vi "PC_Pub_imgFile execution.vi"() -> ()   [LabVIEW 2018]
uses:
  <vilib>/Utility/miscctls.llb/LVRowAndColumnTypeDef.ctl
  <vilib>/nisyscfg/nisyscfg.lvlib
  <resource>/objmgr/nisysapi.rc
  <vilib>/nisyscfg/Close (System).vi
  <vilib>/nisyscfg/Get Installed Components.vi
  QMH/QMH.lvclass
  PC_Pub_imgFile.lvclass
  ProgressBar/ProgressBar.lvclass
  <vilib>/nisyscfg/Create System Image (File).vi
panel:
  in  "Progress":i32(slide) caption="imgDeploy" scale=0.0..100.0
  in  "Retrieve":bool
  in  "Application Image List":string[][](table)
  in  "Deploy":bool
  in  "Target":string(combo)
  out "Current Version":string
  in  "New Version":string
  in  "Description":string
  in  "Title":string
  in  "Image Storage Path":path
  out "Abort":bool
  in  "progressCaption":string
  out "error out":errorcluster
  # "Application Image Properties"
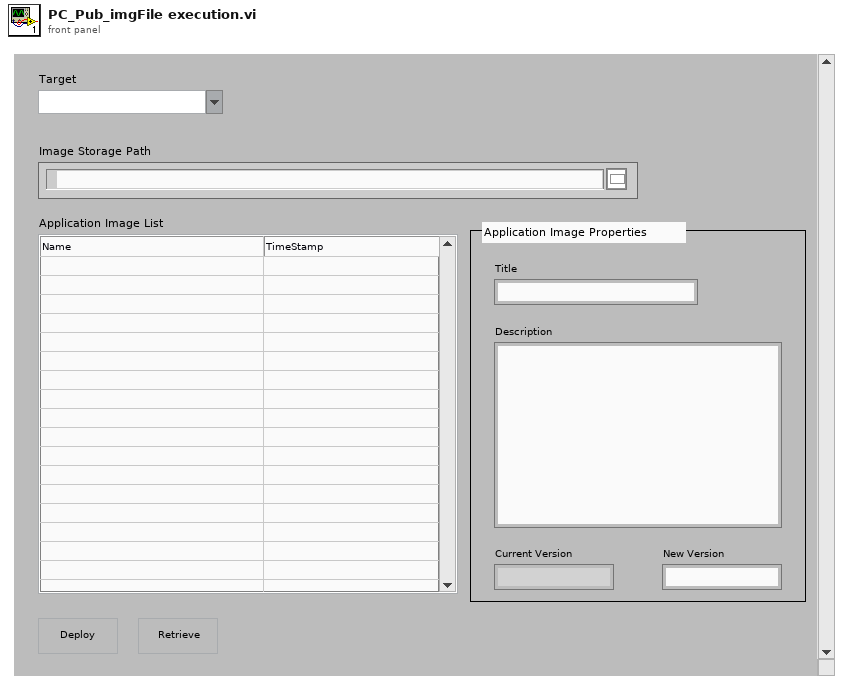
[diagram p1: front panel]
types:
  T1 = typedef "LVRowAndColumnTypeDef.ctl" = cluster{"Row":i32, "Column":i32}
  T2 = cluster{"thisVIRefnum":refnum<vi>, "progressBarRefnum":refnum<vi>, "progressCaption":refnum<vi>}
  T3 = cluster{"Target":refnum<vi>, "Image Storage Path":refnum<vi>, "Pane":refnum<vi>, "Application Image List":refnum<vi>, "Properties":cluster{"Title":refnum<vi>, "Description":refnum<vi>, "Current Version":refnum<vi>, "New Version":refnum<vi>, "id":string}}
  T4 = cluster{"Title":refnum<vi>, "Description":refnum<vi>, "Current Version":refnum<vi>, "New Version":refnum<vi>, "id":string}
  T5 = enum8{"Enabled", "Disabled", "Disabled and Grayed Out"}
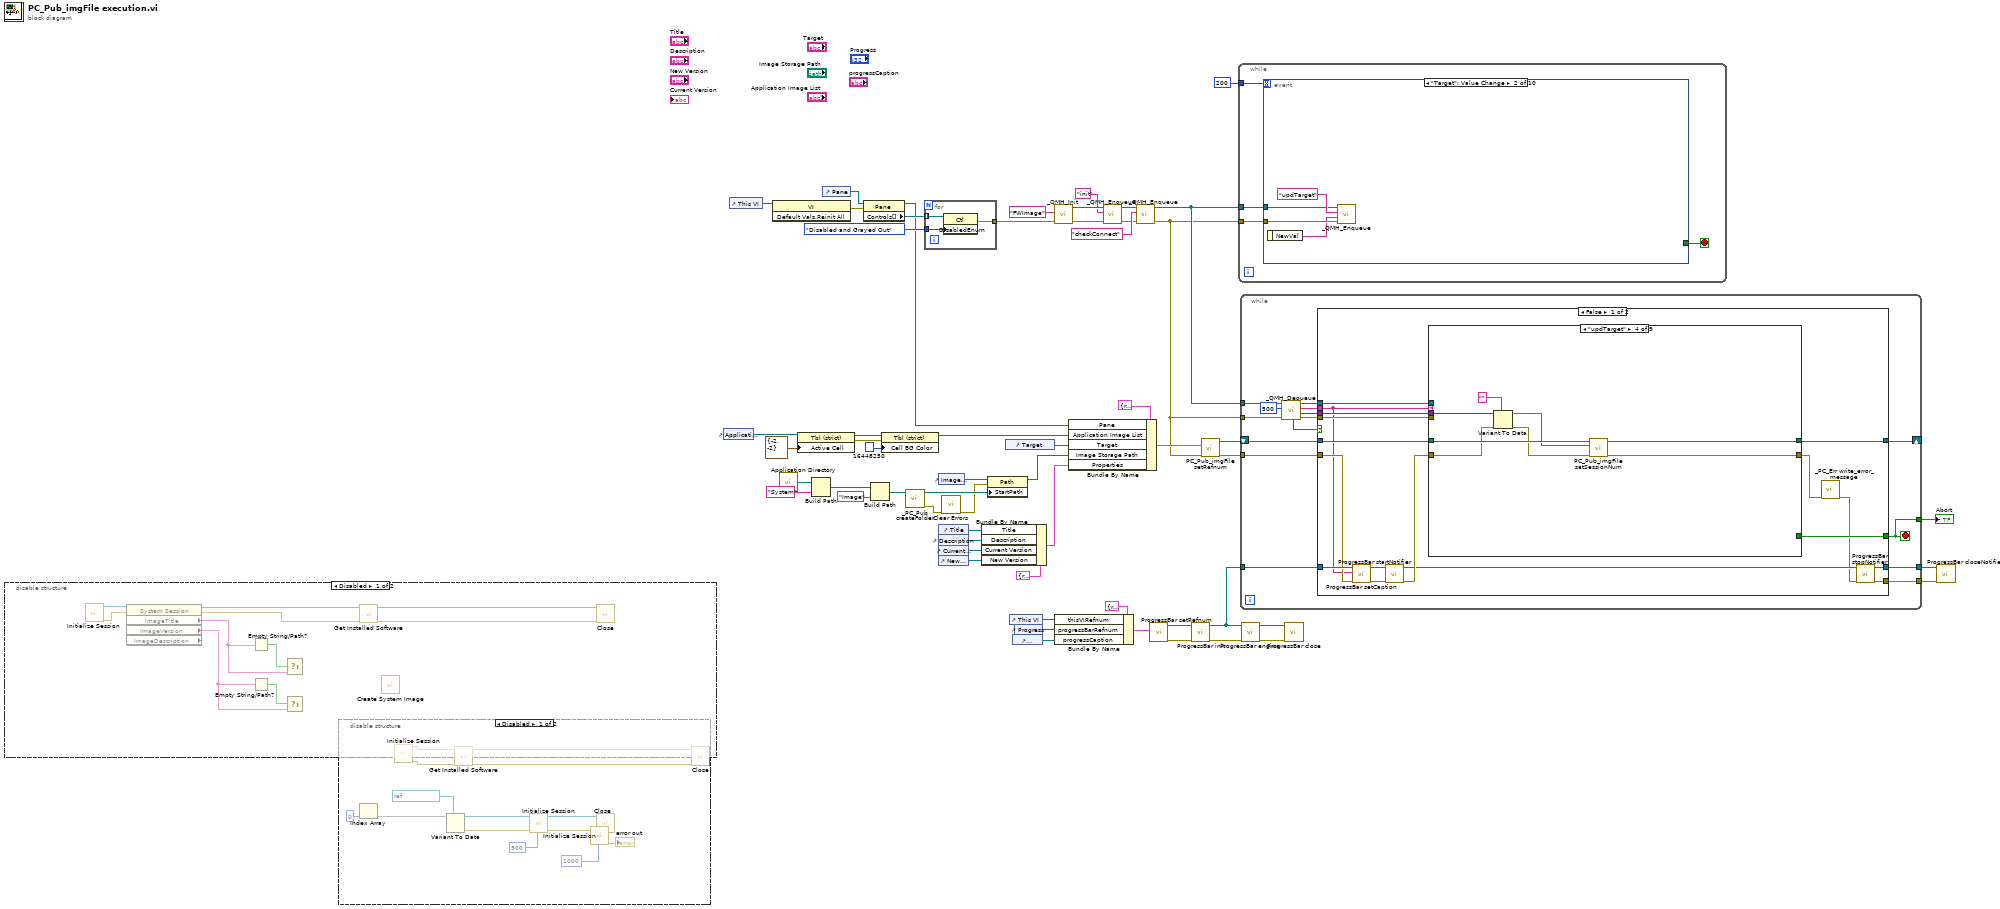
[diagram p0: block diagram]
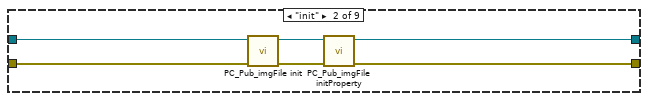
[diagram p3: hidden frame]
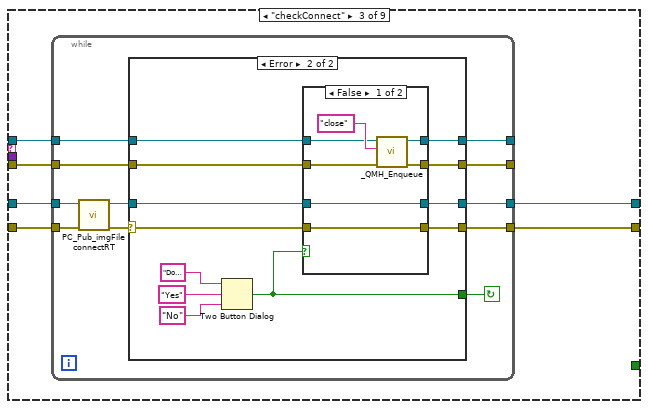
[diagram p4: hidden frame]
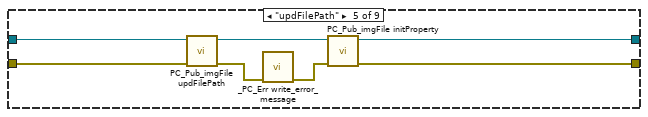
[diagram p7: hidden frame]
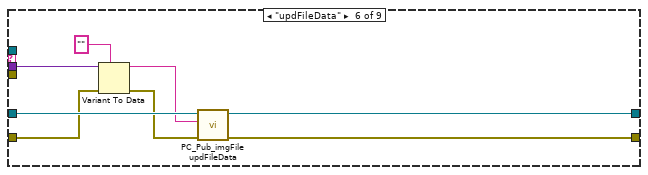
[diagram p8: hidden frame]
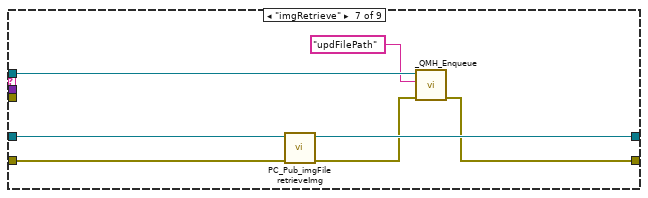
[diagram p9: hidden frame]
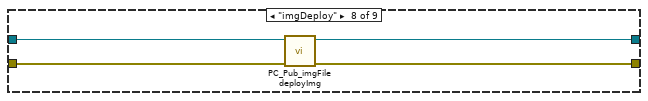
[diagram p10: hidden frame]
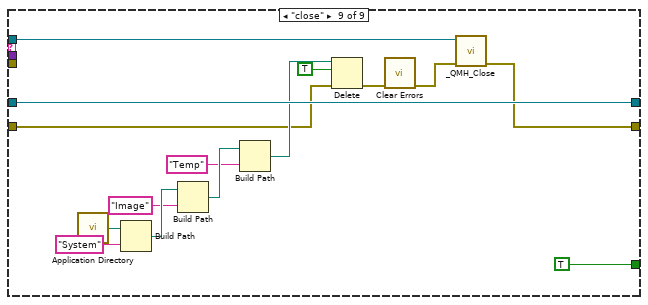
[diagram p11: hidden frame]
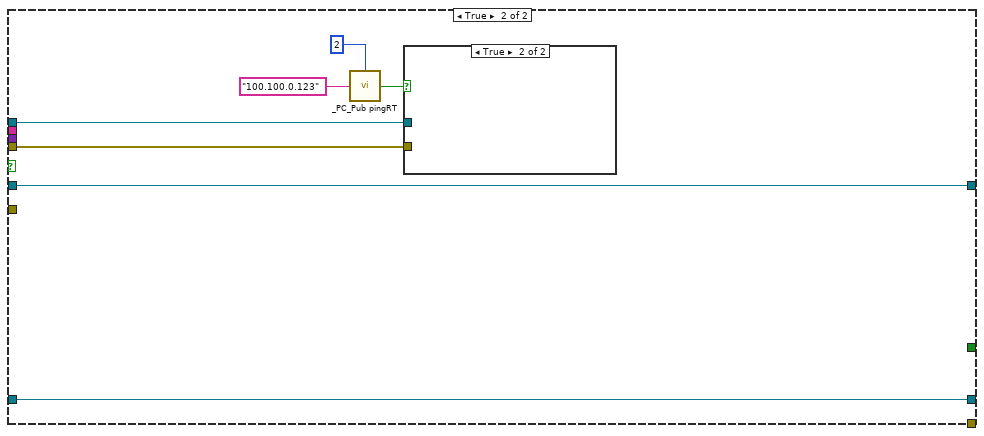
[diagram p12: hidden frame]
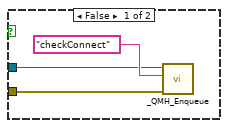
[diagram p13: hidden frame]
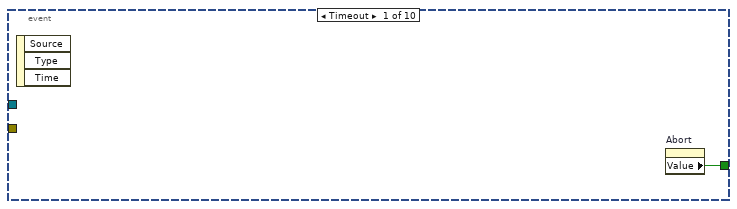
[diagram p14: hidden frame]
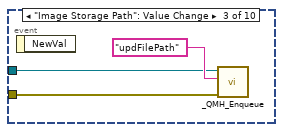
[diagram p15: hidden frame]
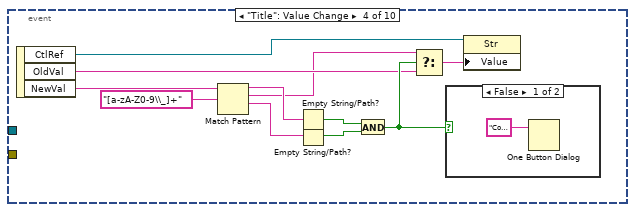
[diagram p16: hidden frame]
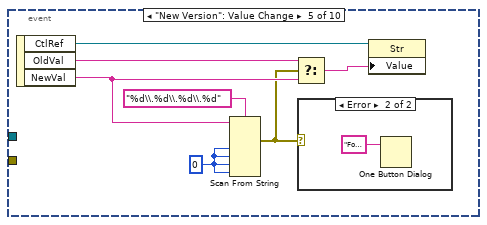
[diagram p18: hidden frame]
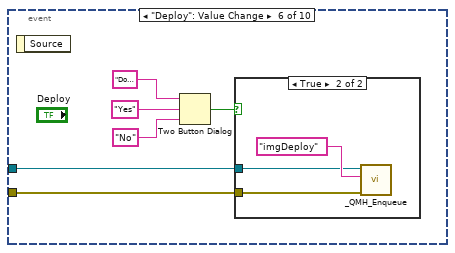
[diagram p20: hidden frame]
diagram:
  n1 = disable-structure shown="Disabled" {
    frame Disabled {
      n2 = call <vilib>:"Initialize Session.vi"() -> ("error out"=w63:errorcluster, "Session out"=w64:refnum<k21>, "Target (localhost)"=w65:refnum<k21>)  [unwired: 9 in]
      n3 = property class="System Session" props=["ImageTitle", "ImageVersion", "ImageDescription"](reference=w64, error in=w63) -> (reference out=w62:refnum<k21>, error out=w61:errorcluster, "ImageTitle"=w69:string, "ImageVersion"=w71:string)  [unwired: 1 out]
      n4 = Empty String/Path?(string/path=w69) -> (empty?=w68:bool)
      n5 = Empty String/Path?(string/path=w71) -> (empty?=w70:bool)
      n6 = Select(s=w68, f=w69) -> (t=w66:string)  [unwired: 1 out]
      n7 = Select(s=w70, f=w71) -> (t=w67:string)  [unwired: 1 out]
      n8 = call-poly <vilib>:"Get Installed Software.vi"("error in (no error)"=w61, "Session in"=w62) -> ("error out"=w59:errorcluster, "Session out"=w60:refnum<k21>)  [unwired: 7 in, 1 out]
      n9 = call-poly <vilib>:"Create System Image.vi"() -> ()  [unwired: 9 in, 3 out]
      n10 = call-poly <vilib>:"Close.vi"("error in (no error)"=w59, "Session in"=w60) -> ()  [unwired: 9 in, 1 out]
    }
    frame Enabled {
    }
  }
  n11 = disable-structure shown="Disabled" {
    frame Disabled {
      n12 = Index Array(index=0) -> (element=w77)  [unwired: 1 in]
      n13 = call <vilib>:"Initialize Session.vi"() -> ("error out"=w84:errorcluster, "Session out"=w85:refnum<k21>, "Target (localhost)"=w80:refnum<k21>)  [unwired: 9 in]
      n14 = Variant To Data(type=refnum<k21> "localhost" ("Target (localhost)"), Variant=w77) -> (data=w76:refnum<k21>, error out=w75:errorcluster)  [unwired: 1 in]
      n15 = call-poly <vilib>:"Get Installed Software.vi"("error in (no error)"=w84, "Session in"=w85) -> ("error out"=w86:errorcluster, "Session out"=w87:refnum<k21>)  [unwired: 7 in, 1 out]
      n16 = call <vilib>:"Initialize Session.vi"("Connect Timeout (4000 ms)"=u32 500, "error in (no error)"=w75, "Target (localhost)"=w76) -> ("error out"=w72:errorcluster, "Session out"=w73:refnum<k21>)  [unwired: 7 in]
      n17 = call <vilib>:"Initialize Session.vi"("Connect Timeout (4000 ms)"=u32 1000) -> ("error out"=→"error out":errorcluster, "Target (localhost)"=w82:refnum<k21>)  [unwired: 8 in, 1 out]
      n18 = call-poly <vilib>:"Close.vi"("error in (no error)"=w72, "Session in"=w73) -> ()  [unwired: 9 in, 1 out]
      n19 = call-poly <vilib>:"Close.vi"("error in (no error)"=w86, "Session in"=w87) -> ()  [unwired: 9 in, 1 out]
    }
    frame Enabled {
    }
  }
  n20 = control-ref of="Application Image List"() -> (w5:refnum<vi>)
  n21 = control-ref of="This VI"() -> (w41:refnum<vi>)
  n22 = invoke class="VI" method="Default Vals.Reinit All"(reference=w41) -> (error out=w40:errorcluster)  [unwired: 2 in, 2 out]
  n23 = call <vilib>:"Application Directory.vi"() -> ("Application Directory"=w38:path)
  n24 = property class="Tbl (strict)"(reference=w5, "Active Cell"=T1 {"Row"=-2, "Column"=-2} ("Active Cell:Active Cell")) -> (reference out=w8:refnum<vi>, error out=w7:errorcluster)  [unwired: 1 in]
  n25 = Build Path(base path=w38, name or relative path="System") -> (appended path=w36:path)
  n26 = control-ref of="Pane"() -> (w57:refnum<vi>)
  n27 = property class="Pane"(reference=w57, error in=w40) -> (reference out=w3:refnum<vi>, "Controls[]"=w56:refnum<vi>[])  [unwired: 1 out]
  n28 = Build Path(base path=w36, name or relative path="Image") -> (appended path=w34:path)
  n29 = property class="Tbl (strict)"(reference=w8, error in=w7, "Cell BG Color"=u32 16448250) -> (reference out=w4:refnum<vi>)  [unwired: 1 out]
  n30 = call "_PC_Pub createFolder.vi"("path (use dialog)"=w34) -> ("error out"=w32:errorcluster, "created path"=w33:path)  [unwired: 9 in]
  n31 = for {
    tunnel: w56 -> [w90] mode=indexing
    tunnel: T5."Disabled and Grayed Out" ("Disabled") -> [w89]
    tunnel: [w88] -> w45
    n32 = property class="Ctl"(reference=w90, "DisabledEnum"=w89) -> (error out=w88:errorcluster)  [unwired: 1 in, 1 out]
  }
  n33 = control-ref of="Title"() -> (w54:refnum<vi>)
  n34 = control-ref of="Description"() -> (w53:refnum<vi>)
  n35 = control-ref of="Current Version"() -> (w52:refnum<vi>)
  n36 = control-ref of="New Version"() -> (w51:refnum<vi>)
  n37 = control-ref of="Image Storage Path"() -> (w43:refnum<vi>)
  n38 = call <vilib>:"Clear Errors.vi"("error in (no error)"=w32) -> ("error out"=w31:errorcluster)  [unwired: 5 in, 1 out]
  n39 = Bundle By Name(cluster=T4 {"Title"=refnum, "Description"=refnum, "Current Version"=refnum, "New Version"=refnum, "id"=""} ("Properties"), "Title"=w54, "Description"=w53, "Current Version"=w52, "New Version"=w51) -> (w42:T4)
  n40 = property class="Path"(reference=w43, error in=w31, "StartPath"=w33) -> (reference out=w39:refnum<vi>)  [unwired: 1 out]
  n41 = control-ref of="Target"() -> (w44:refnum<vi>)
  n42 = control-ref of="This VI"() -> (w17:refnum<vi>)
  n43 = control-ref of="progressCaption"() -> (w15:refnum<vi>)
  n44 = control-ref of="Progress"() -> (w16:refnum<vi>)
  n45 = call "_QMH_Init.vi"("error in (no error)"=w45, "name (unnamed)"="FWImage") -> ("error out"=w29:errorcluster, "QMH out"=w30:refnum<class "QMH.lvclass">)  [unwired: 8 in]
  n46 = Bundle By Name(cluster=T2 {"thisVIRefnum"=refnum, "progressBarRefnum"=refnum, "progressCaption"=refnum} ("refnum"), "thisVIRefnum"=w17, "progressBarRefnum"=w16, "progressCaption"=w15) -> (w14:T2)
  n47 = Bundle By Name(cluster=T3 {"Target"=refnum, "Image Storage Path"=refnum, "Pane"=refnum, "Application Image List"=refnum, "Properties"={"Title"=refnum, "Description"=refnum, "Current Version"=refnum, "New Version"=refnum, "id"=""}} ("refnum"), "Pane"=w3, "Application Image List"=w4, "Target"=w44, "Image Storage Path"=w39, "Properties"=w42) -> (w46:T3)
  n48 = call "_QMH_Enqueue.vi"("error in (no error)"=w29, "Msg"="init", "QMH in"=w30) -> ("error out"=w25:errorcluster, "QMH out"=w26:refnum<class "QMH.lvclass">)  [unwired: 7 in]
  n49 = call "_QMH_Enqueue.vi"("error in (no error)"=w25, "Msg"="checkConnect", "QMH in"=w26) -> ("error out"=w23:errorcluster, "QMH out"=w24:refnum<class "QMH.lvclass">)  [unwired: 7 in]
  n50 = call "ProgressBar setRefnum.vi"("refnum"=w14) -> ("error out"=w21:errorcluster, "ProgressBar out"=w22:refnum<class "ProgressBar.lvclass">)  [unwired: 9 in]
  n51 = call "ProgressBar init.vi"("error in (no error)"=w21, "ProgressBar in"=w22) -> ("error out"=w19:errorcluster, "ProgressBar out"=w20:refnum<class "ProgressBar.lvclass">)  [unwired: 8 in]
  n52 = call "PC_Pub_imgFile setRefnum.vi"("error in (no error)"=w23, "refnum"=w46) -> ("error out"=w48:errorcluster, "imgFile out"=w49:refnum<class "PC_Pub_imgFile.lvclass">)  [unwired: 8 in]
  n53 = while {
    tunnel: w24 -> [w94]
    tunnel: w23 -> [w93]
    tunnel: 200 -> [w91]
    stop <- w92 stop-if-true
    n54 = event shown="[1] \"Target\": Value Change" {
      selector: _ -> [_ _ _ _ _ _ _ _ _ _]
      dyn-events: _ -> [_ _ _ _ _ _ _ _ _ _]
      timeout: w91 -> [_ _ _ _ _ _ _ _ _ _]
      tunnel: w94 -> [_ w98 w101 _ _ w124 w134 _ w149 w165]
      tunnel: w93 -> [_ w97 w100 _ _ w123 w133 _ w148 w164]
      tunnel: [w95 _ _ _ _ _ _ _ _ TRUE] -> w92
      event Timeout {
        n55 = event-data() -> ()  [unwired: 1 in, 3 out]
        n56 = property on="Abort" class="Bool (strict)"() -> ("Value"=w95:bool)  [unwired: 2 in, 2 out]
      }
      event "Target": Value Change {
        n57 = event-data() -> ("NewVal"=w96:string)  [unwired: 1 in]
        n58 = call "_QMH_Enqueue.vi"("error in (no error)"=w97, "Data"=w96, "Msg"="updTarget", "QMH in"=w98) -> ()  [unwired: 6 in, 2 out]
      }
      event "Image Storage Path": Value Change {
        n59 = event-data() -> ()  [unwired: 1 in, 1 out]
        n60 = call "_QMH_Enqueue.vi"("error in (no error)"=w100, "Msg"="updFilePath", "QMH in"=w101) -> ()  [unwired: 7 in, 2 out]
      }
      event "Title": Value Change {
        n61 = event-data() -> ("CtlRef"=w107:refnum<vi>, "OldVal"=w104:string, "NewVal"=w112:string)  [unwired: 1 in]
        n62 = Match Pattern(string=w112, regular expression="[a-zA-Z0-9\\_]+") -> (before substring=w111:string, match substring=w103:string, after substring=w110:string)  [unwired: 1 in, 1 out]
        n63 = Empty String/Path?(string/path=w111) -> (empty?=w109:bool)
        n64 = Empty String/Path?(string/path=w110) -> (empty?=w108:bool)
        n65 = And(x=w109, y=w108) -> (x .and. y?=w105:bool)
        n66 = Select(t=w103, s=w105, f=w104) -> (s? t:f=w106:string)
        n67 = case shown="False" w105 {
          frame False {
            n68 = One Button Dialog(message="Contains incorrect characters") -> ()  [unwired: 1 in, 1 out]
          }
          frame True {
          }
        }
        n69 = property class="Str"(reference=w107, "Value"=w106) -> ()  [unwired: 1 in, 2 out]
      }
      event "New Version": Value Change {
        w121 = u16 0
        n70 = event-data() -> ("CtlRef"=w117:refnum<vi>, "OldVal"=w119:string, "NewVal"=w118:string)  [unwired: 1 in]
        n71 = Scan From String(format string="%d\\.%d\\.%d\\.%d", input string=w118, default 1=w121, default 2=w121, default 3=w121, default 4=w121) -> (error out=w115:errorcluster)  [unwired: 6 in, 2 out]
        n72 = Select(t=w119, s=w115, f=w118) -> (s? t:f=w116:string)
        n73 = case shown="Error" w115 {
          frame No Error {
          }
          frame Error {
            n74 = One Button Dialog(message="Format has error") -> ()  [unwired: 1 in, 1 out]
          }
        }
        n75 = property class="Str"(reference=w117, "Value"=w116) -> ()  [unwired: 1 in, 2 out]
      }
      event "Deploy": Value Change {
        n76 = event-data() -> ()  [unwired: 1 in, 1 out]
        n77 = Two Button Dialog(message="Do you want to deploy system image?", 1:"No" ("F button name (\"Cancel\")"), 2:"Yes" ("T button name (\"OK\")")) -> (T button?=w125:bool)
        n78 = case shown="True" w125 {
          tunnel: w124 -> [_ w130]
          tunnel: w123 -> [_ w129]
          frame False {
          }
          frame True {
            n79 = call "_QMH_Enqueue.vi"("error in (no error)"=w129, "Msg"="imgDeploy", "QMH in"=w130) -> ()  [unwired: 7 in, 2 out]
          }
        }
      }
      event "Retrieve": Value Change {
        n80 = event-data() -> ()  [unwired: 1 in, 1 out]
        n81 = Two Button Dialog(message="Do you want to retrieve system image?", 1:"No" ("F button name (\"Cancel\")"), 2:"Yes" ("T button name (\"OK\")")) -> (T button?=w135:bool)
        n82 = case shown="True" w135 {
          tunnel: w134 -> [_ w139]
          tunnel: w133 -> [_ w138]
          frame False {
          }
          frame True {
            n83 = call "_QMH_Enqueue.vi"("error in (no error)"=w138, "Msg"="imgRetrieve", "QMH in"=w139) -> ()  [unwired: 7 in, 2 out]
          }
        }
      }
      event "Application Image List": Mouse Down? {
        n84 = event-data() -> ("Mods.Double Click"=w142:bool)  [unwired: 1 in]
        n85 = Not(x=w142) -> (.not. x?=w141:bool)
        n86 = event-data("Discard?"=w141) -> ()  [unwired: 1 in, 1 out]
      }
      event "Application Image List": Mouse Down {
        n87 = event-data() -> ("CtlRef"=w156:refnum<vi>)  [unwired: 1 in]
        n88 = property class="Tbl (strict)"(reference=w156) -> (reference out=w155:refnum<vi>, "Value"=w152:string[][], "EditPos"=w153:T1)  [unwired: 1 in, 1 out]
        n89 = Unbundle By Name(w153) -> ("Row"=w143:i32)
        n90 = Index Array(array=w152, index (row)=w143) -> (element=w151:string[])  [unwired: 1 in]
        n91 = property class="Tbl (strict)"(reference=w155, "Key Focus"=FALSE) -> (reference out=w144:refnum<vi>)  [unwired: 1 in, 1 out]
        n92 = Index Array(array=w151, index=0) -> (element=w147:string)
        n93 = Empty String/Path?(string/path=w147) -> (empty?=w146:bool)
        n94 = case shown="False" w146 {
          tunnel: w149 -> [w162 _]
          tunnel: "updFileData" ("Msg") -> [w161 _]
          tunnel: w148 -> [w160 _]
          tunnel: w147 -> [w159 _]
          tunnel: w144 -> [w158 _]
          tunnel: w143 -> [w157 _]
          frame False {
            n95 = call "PC_Pub_imgFile markTableRow.vi"("Row"=w157, "tableRefNum"=w158) -> ()
            n96 = call "_QMH_Enqueue.vi"("error in (no error)"=w160, "Data"=w159, "Msg"=w161, "QMH in"=w162) -> ()  [unwired: 6 in, 2 out]
          }
          frame True {
          }
        }
      }
      event Panel Close {
        n97 = event-data() -> ()  [unwired: 1 in, 1 out]
        n98 = call "_QMH_Enqueue.vi"("error in (no error)"=w164, "Msg"="close", "QMH in"=w165) -> ()  [unwired: 7 in, 2 out]
      }
    }
  }
  n99 = while {
    tunnel: w24 -> [w178]
    tunnel: w48 -> [w180]
    shift-right: [w179] -> _
    shift-left: w49 -> [w181]
    tunnel: w23 -> [w175]
    tunnel: w20 -> [w170]
    tunnel: [w169] -> w13
    tunnel: [w168] -> w12
    tunnel: [w167] -> w1
    stop <- w167 stop-if-true
    n100 = call "_QMH_Dequeue.vi"("error in (no error)"=w175, "timeout in ms (-1)"=500, "QMH in"=w178) -> ("error out"=w173:errorcluster, "Data"=w171:variant, "Msg"=w174:string, "QMH out"=w176:refnum<class "QMH.lvclass">, "timed out?"=w172:bool)  [unwired: 3 in, 1 out]
    n101 = case shown="False" w172 {
      tunnel: w181 -> [w198 w302]
      tunnel: w180 -> [w187 _]
      tunnel: [w197 w302] -> w179
      tunnel: w176 -> [w196 w304]
      tunnel: w174 -> [w184 _]
      tunnel: w173 -> [w195 w303]
      tunnel: [w194 _] -> w167
      tunnel: w171 -> [w193 _]
      tunnel: w170 -> [w188 w301]
      tunnel: [w183 w301] -> w169
      tunnel: [w182 _] -> w168
      frame False {
        n102 = call "ProgressBar setCaption.vi"("error in (no error)"=w187, "newCaption"=w184, "ProgressBar in"=w188) -> ("error out"=w186:errorcluster, "ProgressBar out"=w185:refnum<class "ProgressBar.lvclass">)  [unwired: 7 in]
        n103 = call "ProgressBar startNotifier.vi"("error in (no error)"=w186, "ProgressBar in"=w185) -> ("error out"=w192:errorcluster, "ProgressBar out"=w191:refnum<class "ProgressBar.lvclass">)  [unwired: 8 in]
        n104 = case shown="\"updTarget\"" w184 {
          tunnel: w196 -> [_ _ w208 _ _ _ w277 _ w299]
          tunnel: w198 -> [w200 w206 w212 w258 w265 w273 w280 w284 w298]
          tunnel: w192 -> [w199 w205 w209 w252 w264 w269 w278 w282 w287]
          tunnel: [w200 w202 w211 w257 w262 w272 w279 w283 w298] -> w197
          tunnel: [w199 w201 w210 w256 w261 w266 w275 w281 w297] -> w190
          tunnel: w195 -> [_ _ w207 _ _ _ _ _ _]
          tunnel: [_ _ _ _ _ _ _ _ TRUE] -> w194
          tunnel: w193 -> [_ _ _ w255 _ w271 _ _ _]
          frame Default {
          }
          frame "init" {
            n105 = call "PC_Pub_imgFile init.vi"("error in (no error)"=w205, "imgFile in"=w206) -> ("error out"=w203:errorcluster, "imgFile out"=w204:refnum<class "PC_Pub_imgFile.lvclass">)  [unwired: 8 in]
            n106 = call "PC_Pub_imgFile initProperty.vi"("error in (no error)"=w203, "imgFile in"=w204) -> ("error out"=w201:errorcluster, "imgFile out"=w202:refnum<class "PC_Pub_imgFile.lvclass">)  [unwired: 8 in]
          }
          frame "checkConnect" {
            n107 = while {
              tunnel: w209 -> [w222]
              tunnel: [w215] -> w210
              tunnel: w212 -> [w223]
              tunnel: [w216] -> w211
              tunnel: w208 -> [w218]
              tunnel: w207 -> [w217]
              tunnel: [w214] -> _
              tunnel: [w213] -> _
              stop <- w220 continue-if-true
              n108 = call "PC_Pub_imgFile connectRT.vi"("error in (no error)"=w222, "imgFile in"=w223) -> ("error out"=w221:errorcluster, "imgFile out"=w219:refnum<class "PC_Pub_imgFile.lvclass">)  [unwired: 8 in]
              n109 = case shown="Error" w221 {
                selector: w221 -> [w226 w230]
                tunnel: [_ w236] -> w220
                tunnel: w219 -> [w227 w232]
                tunnel: w218 -> [w225 w235]
                tunnel: w217 -> [w224 w234]
                tunnel: [w227 w233] -> w216
                tunnel: [w226 w231] -> w215
                tunnel: [w225 w229] -> w214
                tunnel: [w224 w228] -> w213
                frame No Error {
                }
                frame Error {
                  n110 = Two Button Dialog(message="Do you want to re-connect", 1:"No" ("F button name (\"Cancel\")"), 2:"Yes" ("T button name (\"OK\")")) -> (T button?=w236:bool)
                  n111 = case shown="False" w236 {
                    tunnel: w235 -> [w245 w248]
                    tunnel: w234 -> [w244 w247]
                    tunnel: [w243 w250] -> w233
                    tunnel: w232 -> [w243 w250]
                    tunnel: [w242 w249] -> w231
                    tunnel: w230 -> [w242 w249]
                    tunnel: [w241 w248] -> w229
                    tunnel: [w240 w247] -> w228
                    frame False {
                      n112 = call "_QMH_Enqueue.vi"("error in (no error)"=w244, "Msg"="close", "QMH in"=w245) -> ("error out"=w240:errorcluster, "QMH out"=w241:refnum<class "QMH.lvclass">)  [unwired: 7 in]
                    }
                    frame True {
                    }
                  }
                }
              }
            }
          }
          frame "updTarget" {
            n113 = Variant To Data(error in=w252, type="", Variant=w255) -> (data=w253:string, error out=w251:errorcluster)
            n114 = call "PC_Pub_imgFile setSessionNum.vi"("error in (no error)"=w251, "newSessionString"=w253, "imgFile in"=w258) -> ("error out"=w256:errorcluster, "imgFile out"=w257:refnum<class "PC_Pub_imgFile.lvclass">)  [unwired: 7 in]
          }
          frame "updFilePath" {
            n115 = call "PC_Pub_imgFile updFilePath.vi"("error in (no error)"=w264, "imgFile in"=w265) -> ("error out"=w260:errorcluster, "imgFile out"=w263:refnum<class "PC_Pub_imgFile.lvclass">)  [unwired: 8 in]
            n116 = call "_PC_Err write_error_message.vi"("error in"=w260) -> ("error out"=w259:errorcluster)  [unwired: 10 in]
            n117 = call "PC_Pub_imgFile initProperty.vi"("error in (no error)"=w259, "imgFile in"=w263) -> ("error out"=w261:errorcluster, "imgFile out"=w262:refnum<class "PC_Pub_imgFile.lvclass">)  [unwired: 8 in]
          }
          frame "updFileData" {
            n118 = Variant To Data(error in=w269, type="", Variant=w271) -> (data=w267:string, error out=w268:errorcluster)
            n119 = call "PC_Pub_imgFile updFileData.vi"("error in (no error)"=w268, "dataName"=w267, "imgFile in"=w273) -> ("error out"=w266:errorcluster, "imgFile out"=w272:refnum<class "PC_Pub_imgFile.lvclass">)  [unwired: 7 in]
          }
          frame "imgRetrieve" {
            n120 = call "PC_Pub_imgFile retrieveImg.vi"("error in (no error)"=w278, "imgFile in"=w280) -> ("error out"=w276:errorcluster, "imgFile out"=w279:refnum<class "PC_Pub_imgFile.lvclass">)  [unwired: 8 in]
            n121 = call "_QMH_Enqueue.vi"("error in (no error)"=w276, "Msg"="updFilePath", "QMH in"=w277) -> ("error out"=w275:errorcluster)  [unwired: 7 in, 1 out]
          }
          frame "imgDeploy" {
            n122 = call "PC_Pub_imgFile deployImg.vi"("error in (no error)"=w282, "imgFile in"=w284) -> ("error out"=w281:errorcluster, "imgFile out"=w283:refnum<class "PC_Pub_imgFile.lvclass">)  [unwired: 8 in]
          }
          frame "close" {
            n123 = call <vilib>:"Application Directory.vi"() -> ("Application Directory"=w294:path)
            n124 = Build Path(base path=w294, name or relative path="System") -> (appended path=w293:path)
            n125 = Build Path(base path=w293, name or relative path="Image") -> (appended path=w295:path)
            n126 = Build Path(base path=w295, name or relative path="Temp") -> (appended path=w288:path)
            n127 = Delete(path (use dialog)=w288, entire hierarchy (F)=TRUE, error in=w287) -> (error out=w286:errorcluster)  [unwired: 2 in, 2 out]
            n128 = call <vilib>:"Clear Errors.vi"("error in (no error)"=w286) -> ("error out"=w285:errorcluster)  [unwired: 5 in, 1 out]
            n129 = call "_QMH_Close.vi"("error in (no error)"=w285, "QMH in"=w299) -> ("error out"=w297:errorcluster)  [unwired: 9 in]
          }
        }
        n130 = call "_PC_Err write_error_message.vi"("error in"=w190) -> ("error out"=w189:errorcluster)  [unwired: 10 in]
        n131 = call "ProgressBar stopNotifier.vi"("error in (no error)"=w189, "ProgressBar in"=w191) -> ("error out"=w182:errorcluster, "ProgressBar out"=w183:refnum<class "ProgressBar.lvclass">)  [unwired: 8 in]
      }
      frame True {
        n132 = call "_PC_Pub pingRT.vi"("IPV4"="100.100.0.123", "items"=2) -> ("valid"=w305:bool)
        n133 = case shown="True" w305 {
          tunnel: w304 -> [w308 _]
          tunnel: w303 -> [w307 _]
          frame False {
            n134 = call "_QMH_Enqueue.vi"("error in (no error)"=w307, "Msg"="checkConnect", "QMH in"=w308) -> ()  [unwired: 7 in, 2 out]
          }
          frame True {
          }
        }
      }
    }
  }
  "Abort" <- w1
  n135 = call "ProgressBar engine.vi"("error in (no error)"=w19, "ProgressBar in"=w20) -> ("error out"=w10:errorcluster, "ProgressBar out"=w11:refnum<class "ProgressBar.lvclass">)  [unwired: 8 in]
  n136 = call "ProgressBar close.vi"("error in (no error)"=w10, "ProgressBar in"=w11) -> ()  [unwired: 8 in, 2 out]
  n137 = call "ProgressBar closeNotifier.vi"("error in (no error)"=w12, "ProgressBar in"=w13) -> ()  [unwired: 8 in, 2 out]
